vi "Is Day Weekend.vi"(11 "Time Stamp":timestamp) -> (3 "weekend?":bool)   [LabVIEW 2018]
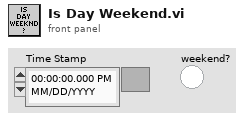
[diagram p1: front panel]
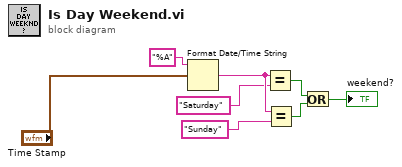
[diagram p0: block diagram]
diagram:
  n1 = Format Date/Time String(time format string (%c)="%A", seconds (now)="Time Stamp") -> (date/time string=w4:string)  [unwired: 1 in]
  n2 = Equal?(x=w4, y="Saturday") -> (x = y?=w7:bool)
  n3 = Equal?(x=w4, y="Sunday") -> (x = y?=w6:bool)
  n4 = Or(x=w7, y=w6) -> (x .or. y?=→"weekend?":bool)
